vi "solar_excel Close.vi"(8 "error in (no error)":errorcluster, 11 "Excel App":T1) -> (0 "error out":errorcluster)   [LabVIEW 2018]
doc: "This closes the Excel application references."
uses:
  solar_excel_ctl App.ctl
  solar_excel_ctl TSV.ctl
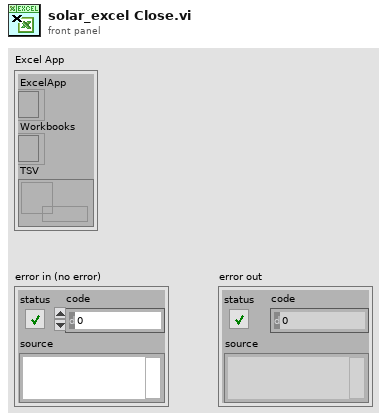
[diagram p1: front panel]
types:
  T1 = typedef "solar_excel_ctl App.ctl" = cluster{"ExcelApp":refnum<k7>, "Workbooks":refnum<k7>, "TSV":refnum<queue>}
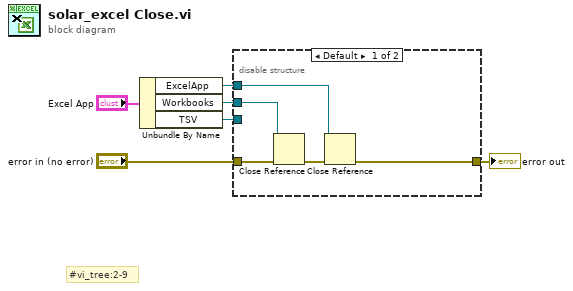
[diagram p0: block diagram]
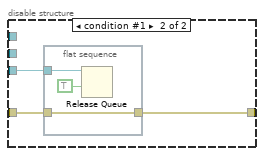
[diagram p2: hidden frame]
diagram:
  # "#vi_tree:2-9"
  n1 = Unbundle By Name("Excel App") -> ("ExcelApp"=w3:refnum<k7>, "Workbooks"=w4:refnum<k7>, "TSV"=w1:refnum<queue>)
  n2 = disable-structure shown="Default" {
    disable-tunnel: "error in (no error)" -> [w11 w12]
    disable-tunnel: w4 -> [w10 _]
    disable-tunnel: w3 -> [w8 _]
    disable-tunnel: [w7 w13] -> w2
    disable-tunnel: w1 -> [_ w14]
    frame condition #0 (active) {
      n3 = Close Reference(reference=w10, error in (no error)=w11) -> (error out=w9:errorcluster)
      n4 = Close Reference(reference=w8, error in (no error)=w9) -> (error out=w7:errorcluster)
    }
    frame condition #1 {
      n5 = flat-sequence {
        tunnel: w14 -> [w17]
        tunnel: [w15] -> w13
        tunnel: w12 -> [w15]
        frame #0 {
          n6 = Release Queue(queue=w17, force destroy? (F)=TRUE) -> ()  [unwired: 1 in, 3 out]
        }
      }
    }
  }
  "error out" <- w2
